vi "CFTS-Show run numbers.vi"(8 "error in (no error)":errorcluster, 11 "Expt State":T1) -> (0 "error out":errorcluster)   [LabVIEW 2020]
doc: "This VI updates the run number indicators on the main Mouse Controller VI. It allows the Mouse Controller display to remain synched with the current state, even when the state is being changed by a measurement VI.\n\nKEH 9/2/09"
uses:
  CFTS-Experiment State.ctl
  CFTS-Globals.vi
panel:
  # "MC-Show run numbers.vi\nThis VI updates the run number indicators on the main Mouse Controller VI. It allows the Mouse Controller display to remain synched with the current state, even when the state is being changed by a measurement VI.\n\nKEH 9/2/09"
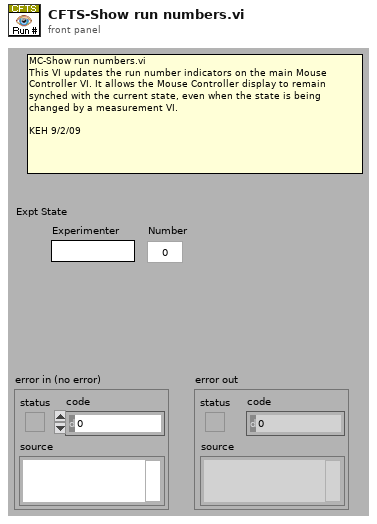
[diagram p1: front panel]
types:
  T1 = typedef "CFTS-Experiment State.ctl" = cluster{"Experimenter":string, "Number":u32, "Right":string, "Left":string, "Data Folder":path, "State File":path, "Version Info":string, "End Exposure Time":dbl, "Exposure Duration":string, "Run #":cluster{"CAP":i16, "ABR":i16, "DP":i16, "VsEP":i16, "MeasSeq":i16, "SubSeq":i16, "SFOAE":i16}}
  T2 = cluster{"CAP RUN #":refnum<vi>, "ABR RUN #":refnum<vi>, "DP RUN #":refnum<vi>, "VsEP RUN #":refnum<vi>}
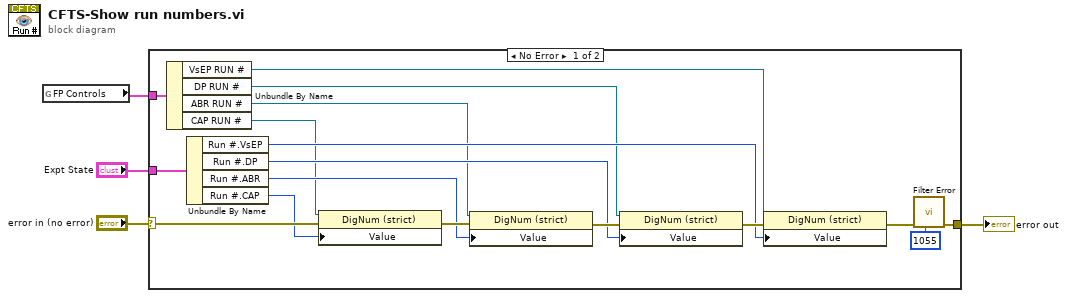
[diagram p0: block diagram]
diagram:
  n1 = global read "CFTS-Globals.vi" "FP Controls"() -> (w2:T2)
  n2 = case shown="No Error" "error in (no error)" {
    selector: "error in (no error)" -> [w20 w22]
    tunnel: [w6 w22] -> w1
    tunnel: "Expt State" -> [w21 _]
    tunnel: w2 -> [w12 _]
    frame No Error {
      n3 = Unbundle By Name(w12) -> ("VsEP RUN #"=w8:refnum<vi>, "DP RUN #"=w9:refnum<vi>, "ABR RUN #"=w10:refnum<vi>, "CAP RUN #"=w11:refnum<vi>)
      n4 = Unbundle By Name(w21) -> ("Run #.VsEP"=w13:i16, "Run #.DP"=w15:i16, "Run #.ABR"=w17:i16, "Run #.CAP"=w19:i16)
      n5 = property class="DigNum (strict)"(reference=w11, error in=w20, "Value"=w19) -> (error out=w18:errorcluster)  [unwired: 1 out]
      n6 = property class="DigNum (strict)"(reference=w10, error in=w18, "Value"=w17) -> (error out=w16:errorcluster)  [unwired: 1 out]
      n7 = property class="DigNum (strict)"(reference=w9, error in=w16, "Value"=w15) -> (error out=w14:errorcluster)  [unwired: 1 out]
      n8 = property class="DigNum (strict)"(reference=w8, error in=w14, "Value"=w13) -> (error out=w7:errorcluster)  [unwired: 1 out]
      n9 = call "Filter Error.vi"("error in (no error)"=w7, "code to ignore"=1055 ("y")) -> ("error out"=w6:errorcluster)  [unwired: 9 in]
    }
    frame Error {
    }
  }
  "error out" <- w1
